vi "Transition.vi"(8 "error in (no error)":errorcluster, 9 "Target State":refnum<class "State.lvclass">, 10 "Source State":refnum<class "State.lvclass">, 11 "External in":refnum<class "External.lvclass">) -> (0 "error out":errorcluster, 2 "State out":refnum<class "State.lvclass">, 3 "External out":refnum<class "External.lvclass">)   [LabVIEW 2024, in "Transition.lvlib" / "External.lvclass"]
uses:
  External.lvclass
  State/State/State.lvclass
  External.lvclass/External.ctl
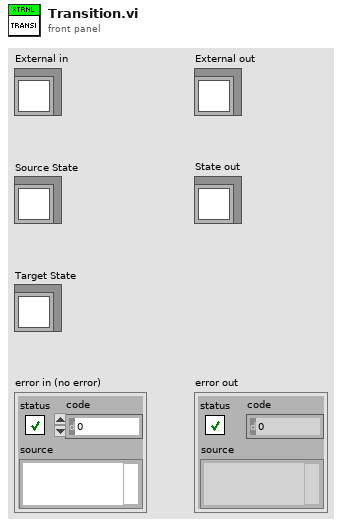
[diagram p1: front panel]
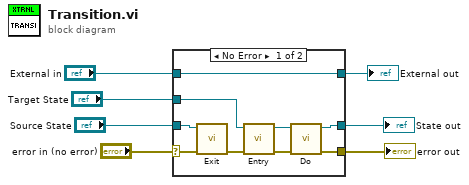
[diagram p0: block diagram]
diagram:
  n1 = case shown="No Error" "error in (no error)" {
    selector: "error in (no error)" -> [w10 w19]
    tunnel: "External in" -> [w9 w18]
    tunnel: [w15 w17] -> w6
    tunnel: [w9 w18] -> w5
    tunnel: [w12 w19] -> w4
    tunnel: "Source State" -> [w11 w17]
    tunnel: "Target State" -> [w8 _]
    frame No Error {
      n2 = call-dynamic "Exit.vi"("error in (no error)"=w10, "State in"=w11) -> ("error out"=w14:errorcluster)  [unwired: 8 in, 1 out]
      n3 = call-dynamic "Entry.vi"("error in (no error)"=w14, "State in"=w8) -> ("error out"=w13:errorcluster, "State out"=w16:refnum<class "State.lvclass">)  [unwired: 8 in]
      n4 = call-dynamic "Do.vi"("error in (no error)"=w13, "State in"=w16) -> ("error out"=w12:errorcluster, "State out"=w15:refnum<class "State.lvclass">)  [unwired: 8 in]
    }
    frame Error {
    }
  }
  "error out" <- w4
  "External out" <- w5
  "State out" <- w6
